vi "TCS_Rx_VISA.vi"() -> ()   [LabVIEW 2018]
uses:
  RxTx/RxTx.lvclass
  Serial Communication/Serial Communication.lvclass
  Serial Communication/Serial Communication.lvclass/Serial Communication.ctl
panel:
  in  "Serial Communication in":refnum<class "Serial Communication.lvclass">
  in  "RxTx.lvclass":refnum<class "RxTx.lvclass">
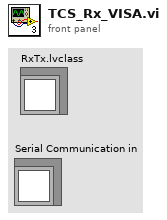
[diagram p1: front panel]
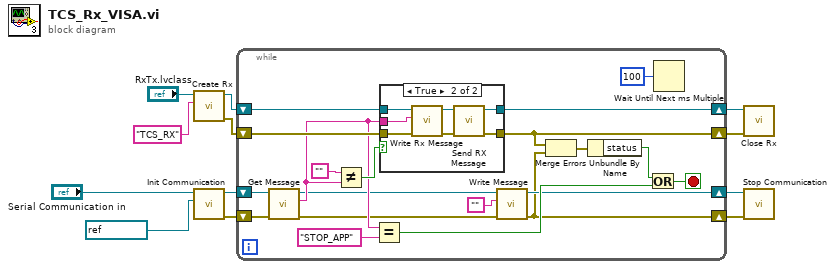
[diagram p0: block diagram]
diagram:
  n1 = call "Create Rx.vi"("Reader Name"="TCS_RX", "RxTx in"="RxTx.lvclass") -> ("error out"=w9:errorcluster, "RxTx out"=w10:refnum<class "RxTx.lvclass">)  [unwired: 8 in]
  n2 = call "Init Communication.vi"("VISA resource name"=refnum<visa-resource-name> "COM2", "Serial Communication in"="Serial Communication in") -> ("error out"=w3:errorcluster, "Serial Communication out"=w4:refnum<class "Serial Communication.lvclass">)  [unwired: 8 in]
  n3 = while {
    shift-right: [w14] -> w1
    shift-left: w3 -> [w21]
    shift-right: [w15] -> w2
    shift-left: w4 -> [w20]
    shift-right: [w28] -> w7
    shift-left: w9 -> [w32]
    shift-right: [w30] -> w8
    shift-left: w10 -> [w31]
    stop <- w24 stop-if-true
    n4 = call "Get Message.vi"("error in (no error)"=w21, "Serial Communication in"=w20) -> ("error out"=w17:errorcluster, "Message"=w19:string, "Serial Communication out"=w18:refnum<class "Serial Communication.lvclass">)  [unwired: 7 in]
    n5 = Not Equal?(x="", y=w19) -> (x != y?=w26:bool)
    n6 = Equal?(x=w19, y="STOP_APP" ("reader name")) -> (x = y?=w22:bool)
    n7 = case shown="True" w26 {
      tunnel: w32 -> [w33 w39]
      tunnel: w31 -> [w34 w38]
      tunnel: w19 -> [_ w37]
      tunnel: [w34 w36] -> w30
      tunnel: [w33 w35] -> w28
      frame False {
      }
      frame True {
        n8 = call "Write Rx Message.vi"("error in (no error)"=w39, "Rx Message"=w37, "RxTx in"=w38) -> ("error out"=w40:errorcluster, "RxTx out"=w41:refnum<class "RxTx.lvclass">)  [unwired: 7 in]
        n9 = call "Send RX Message.vi"("error in (no error)"=w40, "RxTx in"=w41) -> ("error out"=w35:errorcluster, "RxTx out"=w36:refnum<class "RxTx.lvclass">)  [unwired: 8 in]
      }
    }
    n10 = call "Write Message.vi"("error in (no error)"=w17, "Message"="", "Serial Communication in"=w18) -> ("error out"=w14:errorcluster, "Serial Communication out"=w15:refnum<class "Serial Communication.lvclass">)  [unwired: 7 in]
    n11 = Merge Errors(w28, w14) -> (w29:errorcluster)
    n12 = Unbundle By Name(w29) -> ("status"=w23:bool)
    n13 = Or(x=w23, y=w22) -> (x .or. y?=w24:bool)
    n14 = Wait Until Next ms Multiple(millisecond multiple=u32 100 ("milliseconds to wait")) -> ()  [unwired: 1 out]
  }
  n15 = call "Close Rx.vi"("error in (no error)"=w7, "RxTx in"=w8) -> ()  [unwired: 8 in, 2 out]
  n16 = call "Stop Communication.vi"("error in (no error)"=w1, "Serial Communication in"=w2) -> ()  [unwired: 8 in, 2 out]
